vi "verificarDatosRecipe.vi"(8 "error in":errorcluster, 11 "dataToWrite":T2) -> (0 "error out":errorcluster, 3 "dataToWriteModify":T1)   [LabVIEW 2014]
uses:
  <vilib>/addons/database/Auxilliary.llb/DB Tools Format Datetime String (Time Stamp).vi
  <vilib>/addons/database/NI_Database_API.lvlib
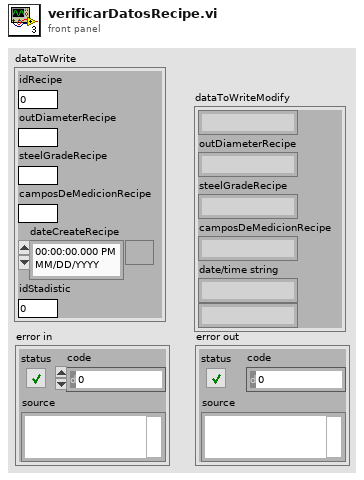
[diagram p1: front panel]
types:
  T1 = cluster{string, "outDiameterRecipe":string, "steelGradeRecipe":string, "camposDeMedicionRecipe":string, "date/time string":string, string}
  T2 = cluster{"idRecipe":dbl, "outDiameterRecipe":string, "steelGradeRecipe":string, "camposDeMedicionRecipe":string, "dateCreateRecipe":timestamp, "idStadistic":dbl}
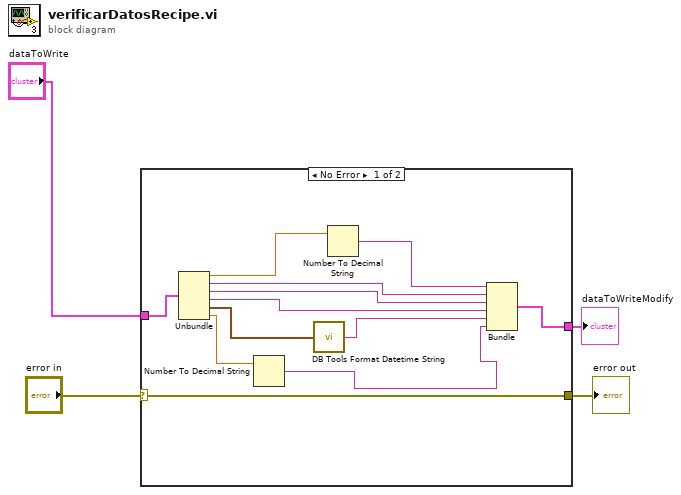
[diagram p0: block diagram]
diagram:
  n1 = case shown="No Error" "error in" {
    selector: "error in" -> [w11 w17]
    tunnel: "dataToWrite" -> [w16 _]
    tunnel: [w15 _] -> w1
    tunnel: [w11 w17] -> w3
    frame No Error {
      n2 = Unbundle(w16) -> ("idRecipe"=w13:dbl, "outDiameterRecipe"=w12:string, "steelGradeRecipe"=w8:string, "camposDeMedicionRecipe"=w7:string, "dateCreateRecipe"=w9:timestamp, "idStadistic"=w6:dbl)
      n3 = Number To Decimal String(number=w6) -> (decimal integer string=w10:string)  [unwired: 1 in]
      n4 = call-poly <vilib>:"DB Tools Format Datetime String.vi"("time stamp"=w9) -> ("date/time string"=w5:string)
      n5 = Number To Decimal String(number=w13) -> (decimal integer string=w14:string)  [unwired: 1 in]
      n6 = Bundle(w14, "outDiameterRecipe"=w12, "steelGradeRecipe"=w8, "camposDeMedicionRecipe"=w7, "date/time string"=w5, w10) -> (w15:T1)  [unwired: 1 in]
    }
    frame Error {
    }
  }
  "error out" <- w3
  "dataToWriteModify" <- w1
